vi "日志报警参数选择 (子VI).vi"(8 "error in (no error)":errorcluster caption="错误输入（无错误）", 11 "String输入":string) -> (0 "error out":errorcluster caption="错误输出", 1 "输出boll数组":bool[](array[boolean]), 2 "输出char数组":string[](array[string]), 3 "输出簇":T1)   [LabVIEW 2016, in "数据传输系统-05.lvlib"]
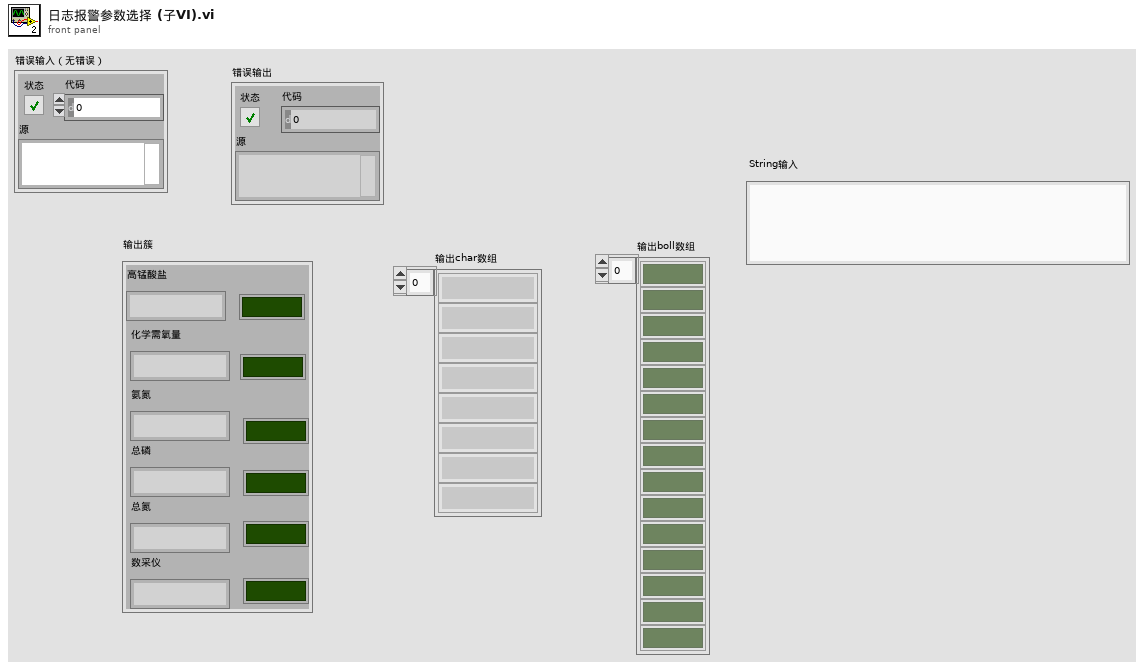
[diagram p1: front panel]
types:
  T1 = cluster{"高锰酸盐":string, "化学需氧量":string, "氨氮":string, "总磷":string, "总氮":string, "数采仪":string, "高锰酸盐":bool, "化学需氧量":bool, "氨氮":bool, "总磷":bool, "总氮":bool, "数采仪":bool}
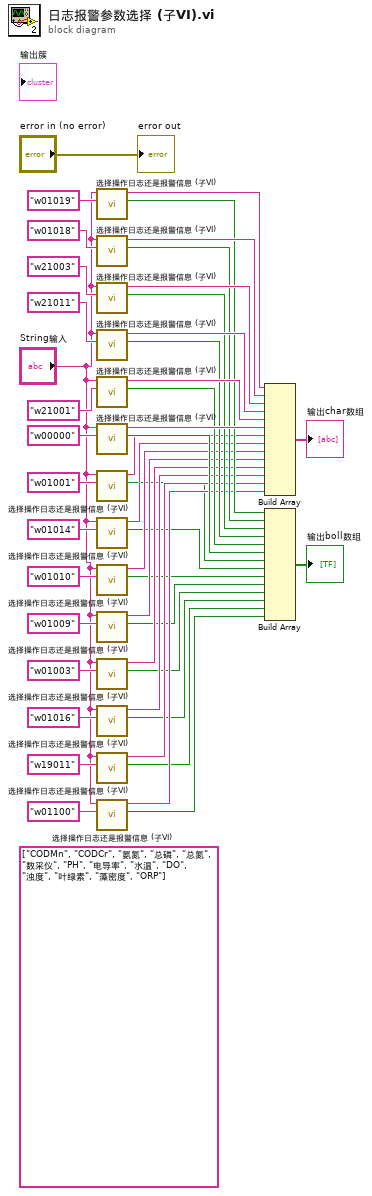
[diagram p0: block diagram]
diagram:
  (unwired) string[] ["CODMn", "CODCr", "氨氮", "总磷", "总氮", "数采仪", "PH", "电导率", "水温", "DO", "浊度", "叶绿素", "藻密度", "ORP"]
  n1 = call "选择操作日志还是报警信息 (子VI).vi"("搜索字符串"="w01019", "Value"="String输入") -> ("布尔"=w32:bool, "名称（未命名）"=w39:string)  [unwired: 8 in]
  n2 = call "选择操作日志还是报警信息 (子VI).vi"("搜索字符串"="w01018", "Value"="String输入") -> ("布尔"=w31:bool, "名称（未命名）"=w38:string)  [unwired: 8 in]
  n3 = call "选择操作日志还是报警信息 (子VI).vi"("搜索字符串"="w21003", "Value"="String输入") -> ("布尔"=w30:bool, "名称（未命名）"=w37:string)  [unwired: 8 in]
  n4 = call "选择操作日志还是报警信息 (子VI).vi"("搜索字符串"="w21011", "Value"="String输入") -> ("布尔"=w29:bool, "名称（未命名）"=w36:string)  [unwired: 8 in]
  n5 = call "选择操作日志还是报警信息 (子VI).vi"("搜索字符串"="w21001", "Value"="String输入") -> ("布尔"=w28:bool, "名称（未命名）"=w35:string)  [unwired: 8 in]
  n6 = call "选择操作日志还是报警信息 (子VI).vi"("搜索字符串"="w00000", "Value"="String输入") -> ("布尔"=w27:bool, "名称（未命名）"=w34:string)  [unwired: 8 in]
  n7 = call "选择操作日志还是报警信息 (子VI).vi"("搜索字符串"="w01001", "Value"="String输入") -> ("布尔"=w9:bool, "名称（未命名）"=w17:string)  [unwired: 8 in]
  n8 = call "选择操作日志还是报警信息 (子VI).vi"("搜索字符串"="w01014", "Value"="String输入") -> ("布尔"=w8:bool, "名称（未命名）"=w16:string)  [unwired: 8 in]
  n9 = call "选择操作日志还是报警信息 (子VI).vi"("搜索字符串"="w01010", "Value"="String输入") -> ("布尔"=w2:bool, "名称（未命名）"=w15:string)  [unwired: 8 in]
  n10 = call "选择操作日志还是报警信息 (子VI).vi"("搜索字符串"="w01009", "Value"="String输入") -> ("布尔"=w3:bool, "名称（未命名）"=w14:string)  [unwired: 8 in]
  n11 = call "选择操作日志还是报警信息 (子VI).vi"("搜索字符串"="w01003", "Value"="String输入") -> ("布尔"=w4:bool, "名称（未命名）"=w13:string)  [unwired: 8 in]
  n12 = call "选择操作日志还是报警信息 (子VI).vi"("搜索字符串"="w01016", "Value"="String输入") -> ("布尔"=w5:bool, "名称（未命名）"=w12:string)  [unwired: 8 in]
  n13 = call "选择操作日志还是报警信息 (子VI).vi"("搜索字符串"="w19011", "Value"="String输入") -> ("布尔"=w6:bool, "名称（未命名）"=w11:string)  [unwired: 8 in]
  n14 = call "选择操作日志还是报警信息 (子VI).vi"("搜索字符串"="w01100", "Value"="String输入") -> ("布尔"=w7:bool, "名称（未命名）"=w10:string)  [unwired: 8 in]
  n15 = Build Array(w39, w38, w37, w36, w35, w34, w17, w16, w15, w14, w13, w12, w11, w10) -> (→"输出char数组":string[])
  n16 = Build Array(w32, w31, w30, w29, w28, w27, w9, w8, w2, w3, w4, w5, w6, w7) -> (→"输出boll数组":bool[])
  "error out" <- "error in (no error)"
